vi "ActiveObjects_DynamicEvents_SendMsgToProcess_5x6x5.vi"(0 "reference in":refnum<class>, 5 "DataToProcess":variant, 11 "Error In":errorcluster) -> (4 "reference out":refnum<class>, 15 "Error Out":errorcluster)   [LabVIEW 2020]
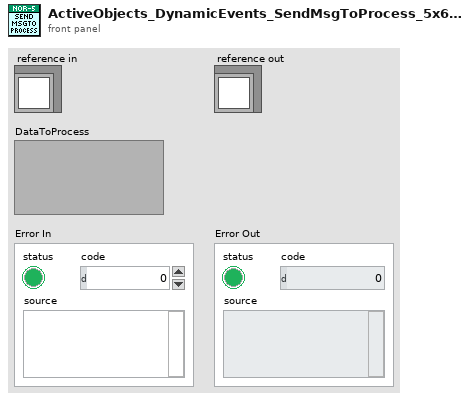
[diagram p1: front panel]
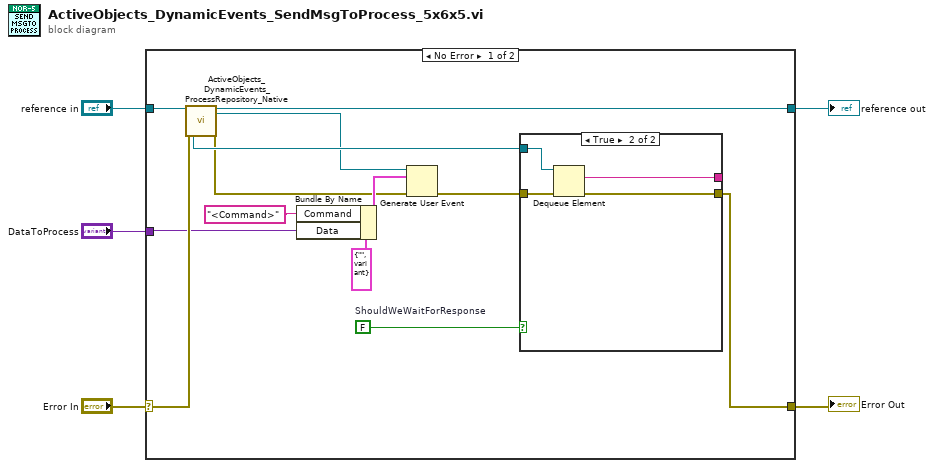
[diagram p0: block diagram]
diagram:
  n1 = case shown="No Error" "Error In" {
    selector: "Error In" -> [w18 w25]
    tunnel: [w8 w25] -> w4
    tunnel: [w16 w24] -> w2
    tunnel: "reference in" -> [w17 w24]
    tunnel: "DataToProcess" -> [w7 _]
    frame No Error {
      w15 = FALSE  # ShouldWeWaitForResponse
      n2 = call <resource>:"ActiveObjects_DynamicEvents_ProcessRepository_Native.vi"("reference in"=w17, "Error In"=w18) -> ("QueueFromProcess"=w11:refnum<queue>, "reference out"=w16:refnum<class>, "EventsToProcess"=w9:refnum<user-event>, "Error Out"=w10:errorcluster)  [unwired: 10 in, 4 out]
      n3 = Bundle By Name(cluster=cluster{"Command":string, "Data":variant} {"Command"="", "Data"=variant} ("MessageToProcess"), "Command"="<Command>", "Data"=w7) -> (w12:cluster{"Command":string, "Data":variant})
      n4 = Generate User Event(user event=w9, event data cluster=w12, error in=w10) -> (error out=w14:errorcluster)  [unwired: 1 in, 1 out]
      n5 = case shown="True" w15 {
        tunnel: w14 -> [w19 w23]
        tunnel: w11 -> [_ w22]
        tunnel: [_ w21] -> _
        tunnel: [w19 w20] -> w8
        frame False {
        }
        frame True {
          n6 = Dequeue Element(queue=w22, error in (no error)=w23) -> (element=w21:string, error out=w20:errorcluster)  [unwired: 1 in, 2 out]
        }
      }
    }
    frame Error {
    }
  }
  "Error Out" <- w4
  "reference out" <- w2
